vi "LABVIEW.vi"() -> ()   [LabVIEW 2020]
uses:
  <vilib>/LabVIEW Interface for Arduino/Type Defs/LCD Pin Config 4 bit.ctl
  <vilib>/LabVIEW Interface for Arduino/LabVIEW Interface for Arduino.lvlib
panel:
  in  "STOP":bool
  in  "Messages":string
  in  "Row":u8
  in  "Column":u8
  in  "LCD Pin Config 4 Bit":T1={"RS"=12, "RW"=255, "Enable"=11, "D4"=5, "D5"=4, "D6"=3, "D7"=2, "LCD"=7}
  in  "VISA resource":refnum<visa-resource-name>
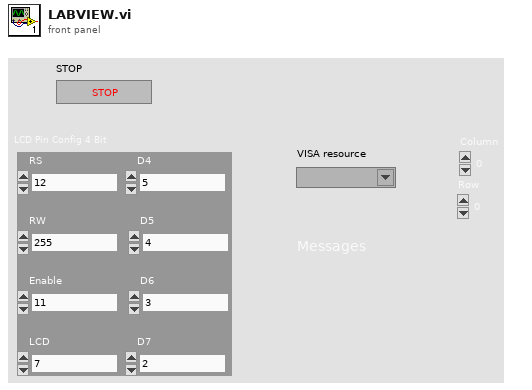
[diagram p1: front panel]
types:
  T1 = typedef "LabVIEW Interface for Arduino.lvlib/LCD Pin Config 4 bit.ctl" = cluster{"RS":u8, "RW":u8, "Enable":u8, "D4":u8, "D5":u8, "D6":u8, "D7":u8, "LCD":u8}
  T2 = typedef "LabVIEW Interface for Arduino.lvlib/Arduino Resource.ctl" = cluster{"VISA resource":refnum<visa-resource-name>, "Board Type":T3, "Connection Type":enum8{"USB / Serial"}, "Bytes Per Packet (15)":u8}
  T3 = typedef "LabVIEW Interface for Arduino.lvlib/Board Type.ctl" = enum16{"Uno", "Dimuelanove w/Atmega 328", "Mega 2560"}
  T4 = enum8{"String", "Binary", "Decimal", "Octal", "Hexadecimal"}
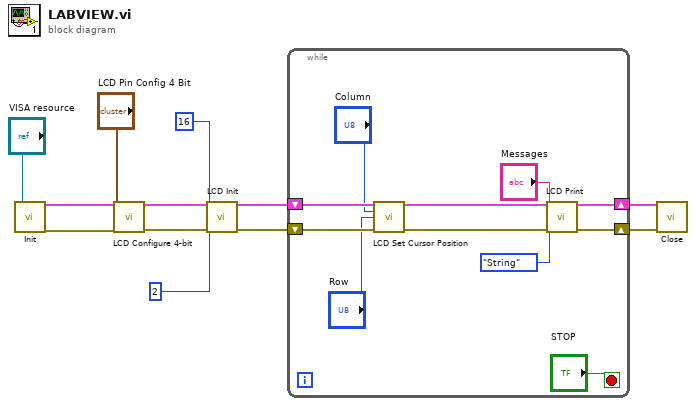
[diagram p0: block diagram]
diagram:
  n1 = call <vilib>:"Init.vi"("VISA resource"="VISA resource") -> ("Arduino Resource"=w12:T2, "error out"=w8:errorcluster)  [unwired: 17 in]
  n2 = call <vilib>:"LCD Configure 4-bit.vi"("Arduino Resource"=w12, "LCD Pin Config 4 Bit"="LCD Pin Config 4 Bit", "error in"=w8) -> ("Arduino Resource"=w11:T2, "error out"=w7:errorcluster)  [unwired: 11 in]
  n3 = call <vilib>:"LCD Init.vi"("Arduino Resource"=w11, "Columns"=u8 16, "Rows"=u8 2, "error in"=w7) -> ("Arduino Resource"=w10:T2, "error out"=w6:errorcluster)  [unwired: 10 in]
  n4 = while {
    shift-right: [w21] -> w9
    shift-left: w10 -> [w23]
    shift-right: [w18] -> w5
    shift-left: w6 -> [w20]
    stop <- "STOP" stop-if-true
    n5 = call <vilib>:"LCD Set Cursor Position.vi"("Arduino Resource"=w23, "Column"="Column", "Row"="Row", "error out"=w20) -> ("Arduino Resource"=w22:T2, "error out"=w19:errorcluster)  [unwired: 10 in]
    n6 = call <vilib>:"LCD Print.vi"("Arduino Resource"=w22, "Data"="Messages", "Base (String)"=T4."String", "error out"=w19) -> ("Arduino Resource"=w21:T2, "error out"=w18:errorcluster)  [unwired: 10 in]
  }
  n7 = call <vilib>:"Close.vi"("Arduino Resource"=w9, "error in"=w5) -> ()  [unwired: 13 in, 1 out]
